vi "ligar_forno(SubVI).vi"(8 "error in (no error)":errorcluster, 10 "s":bool, 11 "VISA Refnum in":refnum<visa-resource-name>) -> (0 "error out":errorcluster, 3 "VISA resource name out":refnum<visa-resource-name>)   [LabVIEW 2018]
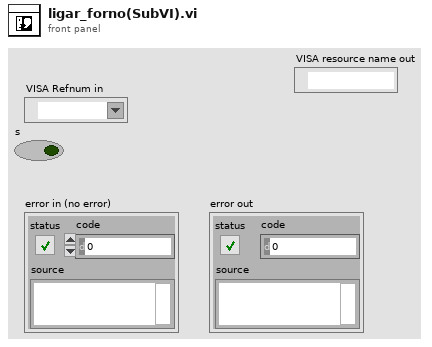
[diagram p1: front panel]
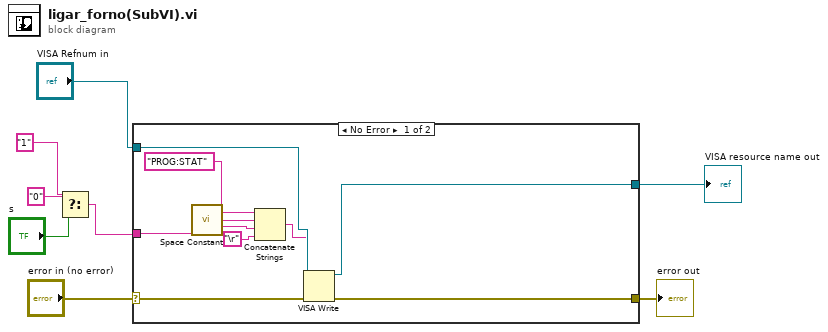
[diagram p0: block diagram]
diagram:
  n1 = Select(t="1", s="s", f="0") -> (s? t:f=w5:string)
  n2 = case shown="No Error" "error in (no error)" {
    selector: "error in (no error)" -> [w11 w19]
    tunnel: [w17 w19] -> w8
    tunnel: "VISA Refnum in" -> [w16 w18]
    tunnel: w5 -> [w10 _]
    tunnel: [w9 w18] -> w1
    frame No Error {
      n3 = call <vilib>:"Space Constant.vi"() -> ("String"=w14:string)
      n4 = Concatenate Strings("PROG:STAT" ("string"), w14, w10, "\r") -> (w15:string)
      n5 = VISA Write(VISA resource name=w16, write buffer=w15, error in (no error)=w11) -> (VISA resource name out=w9:refnum<visa-resource-name>, error out=w17:errorcluster)  [unwired: 1 out]
    }
    frame Error {
    }
  }
  "error out" <- w8
  "VISA resource name out" <- w1
